vi "Close_Redis.vi"(0 "Refnum in":refnum<vi>, 11 "error in":errorcluster) -> (4 "Refnum out":refnum<vi>, 6 "Data":T1, 8 "Connection Closed ?":bool, 15 "error out":errorcluster)   [LabVIEW 2020]
uses:
  SubVIs/Controls/redis-data.ctl
  Redis Commands/Connection/QUIT.vi
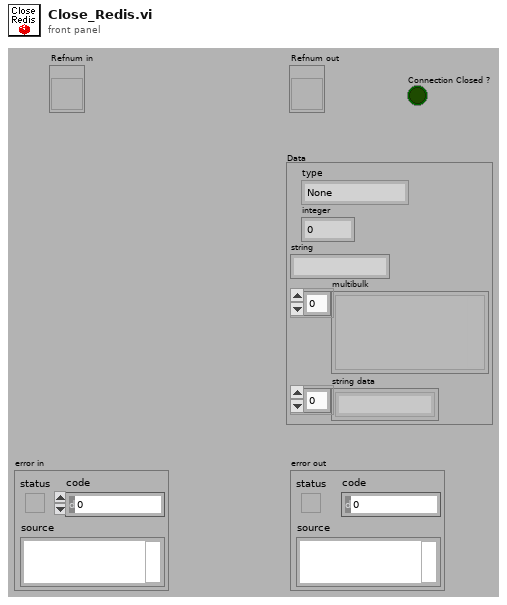
[diagram p1: front panel]
types:
  T1 = typedef "redis-data.ctl" = cluster{"type":enum16{"None", "Error", "Status", "Nil", "Integer", "String", "Multibulk"}, "integer":i64, "string":string, "multibulk":variant[], "string data":string[]}
  T2 = enum16{"None", "Error", "Status", "Nil", "Integer", "String", "Multibulk"}
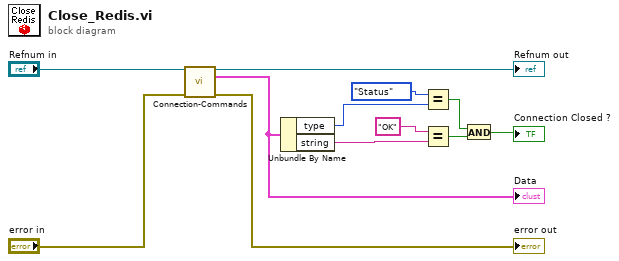
[diagram p0: block diagram]
diagram:
  n1 = call-poly "Connection-Commands.vi"("refnum in"="Refnum in", "error in"="error in") -> ("refnum out"=→"Refnum out":refnum<vi>, "Data"=w1:T1, "error out"=→"error out":errorcluster)  [unwired: 11 in]
  "Data" <- w1
  n2 = Unbundle By Name(w1) -> ("type"=w5:T2, "string"=w7:string)
  n3 = Equal?(x=T2."Status" ("type"), y=w5) -> (x = y?=w10:bool)
  n4 = Equal?(x="OK", y=w7) -> (x = y?=w9:bool)
  n5 = And(x=w10, y=w9) -> (x .and. y?=→"Connection Closed ?":bool)
